vi "VISA_Read.vi"(8 "Error":errorcluster caption="错误输入（无错误）", 10 "字节总数":u32=10, 11 "VISA resource name":refnum<visa-resource-name>) -> (0 "Error out":errorcluster, 2 "读取缓冲区":string, 3 "VISA resource name out":refnum<visa-resource-name>)   [LabVIEW 2020]
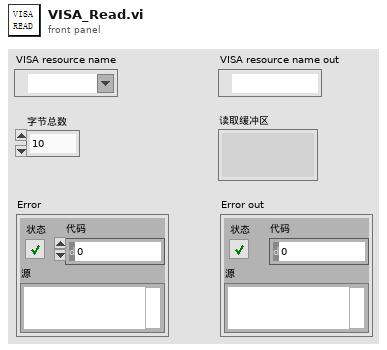
[diagram p1: front panel]
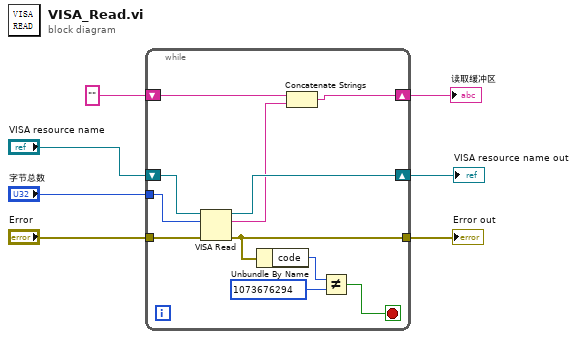
[diagram p0: block diagram]
diagram:
  n1 = while {
    tunnel: "字节总数" -> [w17]
    tunnel: "Error" -> [w16]
    shift-right: [w13] -> w2
    shift-left: "VISA resource name" -> [w18]
    shift-right: [w10] -> w3
    shift-left: "" -> [w12]
    tunnel: [w8] -> w1
    stop <- w9 stop-if-true
    n2 = VISA Read(VISA resource name=w18, byte count=w17, error in (no error)=w16) -> (VISA resource name out=w13:refnum<visa-resource-name>, read buffer=w11:string, error out=w8:errorcluster)  [unwired: 1 out]
    n3 = Unbundle By Name(w8) -> ("code"=w15:i32)
    n4 = Concatenate Strings(w12, w11) -> (w10:string)
    n5 = Not Equal?(x=w15, y=1073676294) -> (x != y?=w9:bool)
  }
  "VISA resource name out" <- w2
  "Error out" <- w1
  "读取缓冲区" <- w3
